vi "Close DCAF INI.vi"(8 "Error In":errorcluster) -> (0 "Error Out":errorcluster)   [LabVIEW 2014, in "Standard Editor.lvlib" / "DCAF INI.lvlib"]
doc: "Close reference to DCAF INI file."
uses:
  DCAF INI.lvlib
  <vilib>/Utility/config.llb/NI_LVConfig.lvlib
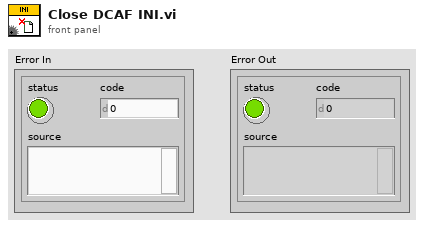
[diagram p1: front panel]
types:
  T1 = typedef "NI_LVConfig.lvlib/Config Data RefNum.ctl" = refnum<k1>
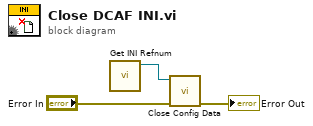
[diagram p0: block diagram]
diagram:
  n1 = call "Get INI Refnum.vi"() -> ("INI Refnum Out"=w1:T1)  [unwired: 11 in]
  n2 = call <vilib>:"Close Config Data.vi"("error in (no error)"="Error In", "refnum"=w1) -> ("error out"=→"Error Out":errorcluster)  [unwired: 8 in, 1 out]
